vi "svfa_Check for AvgParam Change (Dual).vi"(4 "measurement":T1(ring), 6 "averaging parameters":T2={"averaging mode"=enum."No averaging", "weighting mode"=enum."Linear", "number of averages"=10, "linear mode"=enum."Auto restart"}, 7 "restart averaging (F)":bool, 8 "error in (no error)":errorcluster) -> (0 "error out":errorcluster, 1 "parameter has changed":bool)   [LabVIEW 2017]
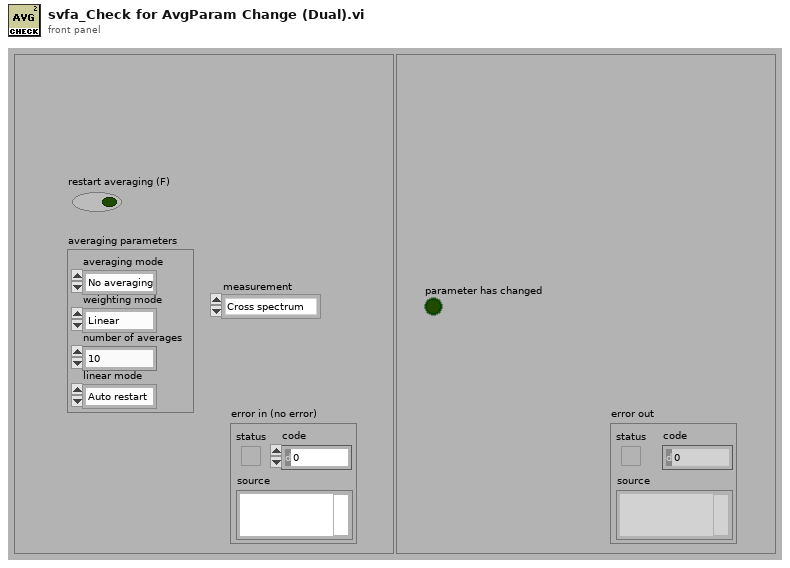
[diagram p1: front panel]
types:
  T1 = enum16{"Cross spectrum", "Frequency response", "Coherent output power"}
  T2 = cluster{"averaging mode":enum16{"No averaging", "Vector averaging", "RMS averaging", "Peak hold"}, "weighting mode":enum16{"Linear", "Exponential"}, "number of averages":u32, "linear mode":enum16{"One shot", "Auto restart"}}
  T3 = enum16{"No averaging", "Vector averaging", "RMS averaging", "Peak hold"}
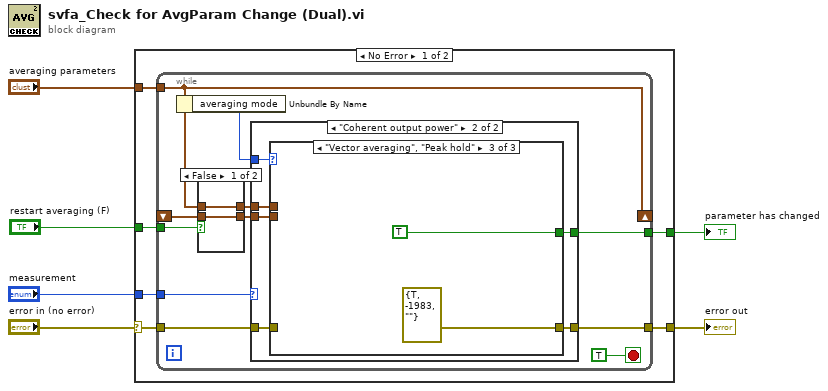
[diagram p0: block diagram]
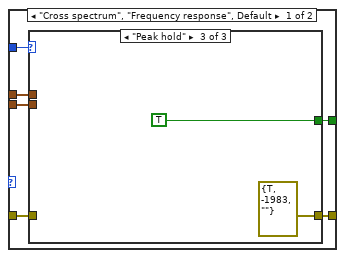
[diagram p3: hidden frame]
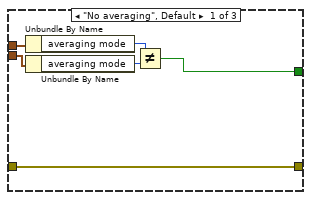
[diagram p4: hidden frame]
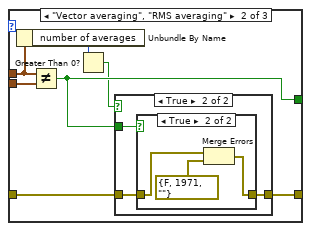
[diagram p5: hidden frame]
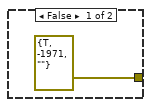
[diagram p6: hidden frame]
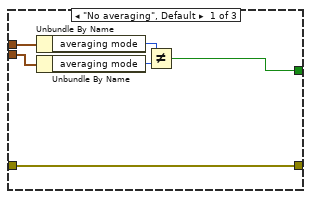
[diagram p8: hidden frame]
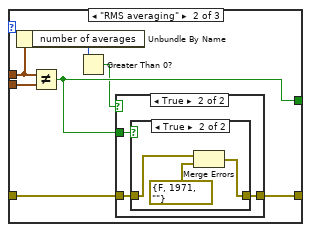
[diagram p9: hidden frame]
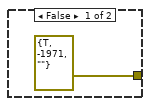
[diagram p10: hidden frame]
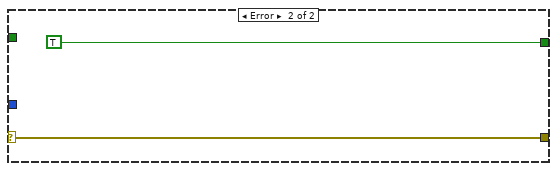
[diagram p12: hidden frame]
diagram:
  n1 = case shown="No Error" "error in (no error)" {
    selector: "error in (no error)" -> [w9 w86]
    tunnel: [w8 w86] -> w5
    tunnel: "averaging parameters" -> [w12 _]
    tunnel: [w11 TRUE] -> w4
    tunnel: "measurement" -> [w10 _]
    tunnel: "restart averaging (F)" -> [w7 _]
    frame No Error {
      n2 = while {
        tunnel: [w18] -> w8
        tunnel: w9 -> [w19]
        tunnel: w10 -> [w20]
        tunnel: [w22] -> w11
        tunnel: w12 -> [w16]
        shift-left: _ -> [w14]
        shift-right: [w16] -> _
        tunnel: w7 -> [w13]
        stop <- TRUE stop-if-true
        n3 = Unbundle By Name(w16) -> ("averaging mode"=w21:T3)
        n4 = case shown="False" w13 {
          tunnel: w16 -> [w24 w26]
          tunnel: [w24 w26] -> w17
          tunnel: [w25 w26] -> w15
          tunnel: w14 -> [w25 _]
          frame False {
          }
          frame True {
          }
        }
        n5 = case shown="\"Coherent output power\"" w20 {
          tunnel: w15 -> [w27 w59]
          tunnel: [w32 w58] -> w22
          tunnel: w21 -> [w31 w61]
          tunnel: w17 -> [w30 w60]
          tunnel: w19 -> [w29 w56]
          tunnel: [w28 w57] -> w18
          frame "Cross spectrum", "Frequency response", Default {
            n6 = case shown="\"Peak hold\"" w31 {
              tunnel: w30 -> [w37 w44 _]
              tunnel: w27 -> [w36 w45 _]
              tunnel: [w33 w41 TRUE] -> w32
              tunnel: w29 -> [w38 w42 _]
              tunnel: [w38 w40 errorcluster {"status"=TRUE, "code"=-1983, "source"=""} ("error IO")] -> w28
              frame "No averaging", Default {
                n7 = Unbundle By Name(w37) -> ("averaging mode"=w34:T3)
                n8 = Unbundle By Name(w36) -> ("averaging mode"=w35:T3)
                n9 = Not Equal?(x=w34, y=w35) -> (x != y?=w33:bool)
              }
              frame "Vector averaging", "RMS averaging" {
                n10 = Unbundle By Name(w44) -> ("number of averages"=w43:u32)
                n11 = Not Equal?(x=w44, y=w45) -> (x != y?=w41:bool)
                n12 = Greater Than 0?(x=w43) -> (x > 0?=w39:bool)
                n13 = case shown="True" w39 {
                  tunnel: w42 -> [_ w49]
                  tunnel: w41 -> [_ w48]
                  tunnel: [errorcluster {"status"=TRUE, "code"=-1971, "source"=""} ("error IO") w47] -> w40
                  frame False {
                  }
                  frame True {
                    n14 = case shown="True" w48 {
                      tunnel: [w50 w51] -> w47
                      tunnel: w49 -> [w50 w53]
                      frame False {
                      }
                      frame True {
                        n15 = Merge Errors(w53, errorcluster {"status"=FALSE, "code"=1971, "source"=""} ("error IO")) -> (w51:errorcluster)
                      }
                    }
                  }
                }
              }
              frame "Peak hold" {
              }
            }
          }
          frame "Coherent output power" {
            n16 = case shown="\"Vector averaging\", \"Peak hold\"" w61 {
              tunnel: w60 -> [w64 w73 _]
              tunnel: w59 -> [w63 w74 _]
              tunnel: [w62 w69 TRUE] -> w58
              tunnel: [w67 w70 errorcluster {"status"=TRUE, "code"=-1983, "source"=""} ("error IO")] -> w57
              tunnel: w56 -> [w67 w71 _]
              frame "No averaging", Default {
                n17 = Unbundle By Name(w64) -> ("averaging mode"=w65:T3)
                n18 = Unbundle By Name(w63) -> ("averaging mode"=w66:T3)
                n19 = Not Equal?(x=w65, y=w66) -> (x != y?=w62:bool)
              }
              frame "RMS averaging" {
                n20 = Unbundle By Name(w73) -> ("number of averages"=w72:u32)
                n21 = Not Equal?(x=w73, y=w74) -> (x != y?=w69:bool)
                n22 = Greater Than 0?(x=w72) -> (x > 0?=w68:bool)
                n23 = case shown="True" w68 {
                  tunnel: w71 -> [_ w78]
                  tunnel: [errorcluster {"status"=TRUE, "code"=-1971, "source"=""} ("error IO") w77] -> w70
                  tunnel: w69 -> [_ w76]
                  frame False {
                  }
                  frame True {
                    n24 = case shown="True" w76 {
                      tunnel: [w79 w80] -> w77
                      tunnel: w78 -> [w79 w82]
                      frame False {
                      }
                      frame True {
                        n25 = Merge Errors(w82, errorcluster {"status"=FALSE, "code"=1971, "source"=""} ("error IO")) -> (w80:errorcluster)
                      }
                    }
                  }
                }
              }
              frame "Vector averaging", "Peak hold" {
              }
            }
          }
        }
      }
    }
    frame Error {
    }
  }
  "error out" <- w5
  "parameter has changed" <- w4
